vi "getFirstNumber.vi"(8 "error in (no error)":errorcluster, 11 "View in":refnum<class "View.lvclass">) -> (0 "error out":errorcluster, 2 "firstNumber":dbl, 3 "View out":refnum<class "View.lvclass">)   [LabVIEW 2016, in "View.lvclass"]
uses:
  View.lvclass
  View.lvclass/View.ctl
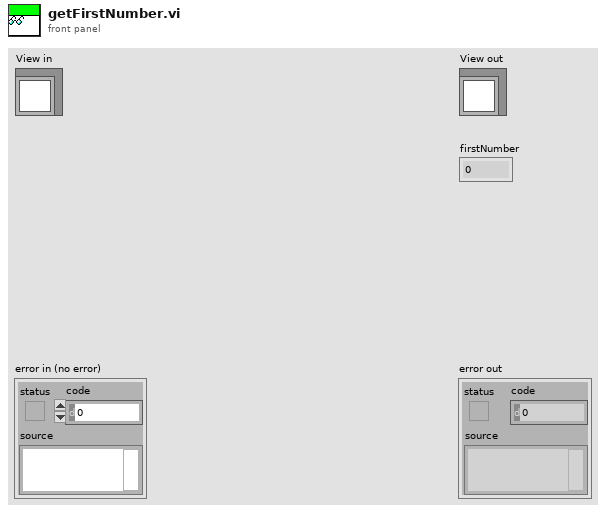
[diagram p1: front panel]
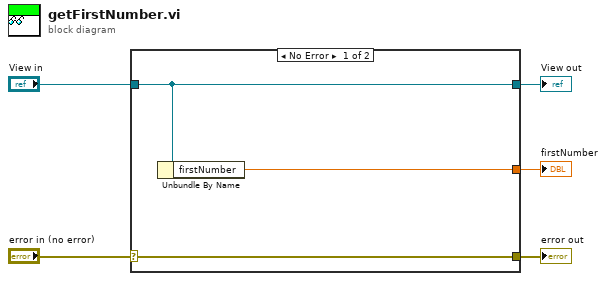
[diagram p0: block diagram]
diagram:
  n1 = case shown="No Error" "error in (no error)" {
    selector: "error in (no error)" -> [w8 w9]
    tunnel: [w8 w9] -> w4
    tunnel: [w7 w10] -> w2
    tunnel: "View in" -> [w7 w10]
    tunnel: [w6 _] -> w1
    frame No Error {
      n2 = Unbundle By Name(w7) -> ("firstNumber"=w6:dbl)
    }
    frame Error {
    }
  }
  "error out" <- w4
  "View out" <- w2
  "firstNumber" <- w1
